vi "instrument_detector.vi"() -> ()   [LabVIEW 2018]
panel:
  out "error in (no error) 2":errorcluster
  in  "error in (no error)":errorcluster
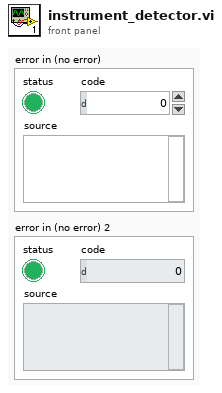
[diagram p1: front panel]
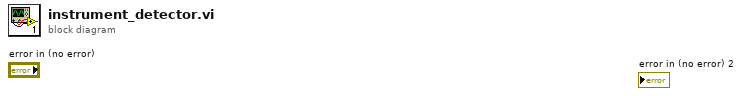
[diagram p0: block diagram]
diagram:
